vi "AppliedMotionDriveParams.vi"(4 "queue out":refnum<queue>, 6 "user event out":refnum<user-event>, 8 "error in (no error)":errorcluster, 11 "AppliedMotionDrive.lvclass":refnum<class "AppliedMotionDrive.lvclass">) -> (0 "error out":errorcluster, 3 "AppliedMotionDrive.lvclass Out":refnum<class "AppliedMotionDrive.lvclass">)   [LabVIEW 2019, in "AppliedMotionDrive.lvclass"]
doc: "Ce VI est une interface utilisateur qui permet à l'usager d'interagir avec le contrôlleur de moteur ST5-Q"
uses:
  AppliedMotionDrive.lvclass
  C:/Programmes Labview/LabscanV1A/DevicesClass/BaseDevice/BaseDevice.lvclass
  <vilib>/Utility/error.llb/DialogType.ctl
  AppliedMotionDrive.lvclass/AppliedMotionDrive.ctl
panel:
  in  "Update Instr":bool
  in  "Save Act":bool
  in  "LoadAct":bool
  in  "Actuator Settings":u16(ring) items=["Sample Wheel", "Photolum Height", "Filter Wheel"]
  in  "Units":u16(ring) items=["mm", "deg", "pas", "holes"]
  out "Instrument Name":string
  in  "Init":bool
  out "CW Limit":bool
  out "CCW Limit":bool
  out "Alarme":u32
  in  "Update":bool
  in  "Clr Alarm":bool
  out "Status":T1
  in  "Résolution Pas":dbl
  in  "Facteur Dir":bool
  in  "Facteur Pas":dbl=1500.0
  in  "Save":bool
  in  "Accél Max":dbl=0.167 caption="Accélération Max (Tour/s/s)" min=0.167 max=5461.167 step=0.167 format="%#.3g"
  in  "Stop":bool
  in  "Relatif":bool=TRUE caption="Relatif/Absolu\n(Absolu)"
  in  "Origine":bool
  in  "Direction":bool=TRUE
  in  "Déplacement":dbl caption="Position (holes)" min=-2000.0 max=2000.0 step=0.0001 format="%#.3g"
  in  "Décél":dbl=0.167 caption="Décélération \n(Tour/s/s)" min=0.167 max=5461.167 step=0.167 format="%#.3g"
  in  "Accél":dbl=0.167 caption="Accélération \n(Tour/s/s)" min=0.167 max=5461.167 step=0.167 format="%#.3g"
  out "Réponse":string
  in  "Commande":string
  out "Port COM":refnum<visa-resource-name>="COM4"
  in  "Envoyer":bool
  in  "Vitesse":dbl=0.08399999999999999 caption="Vitesse (Tour/s)" min=0.0042 max=133.3333 step=0.0042 format="%#.4g"
  in  "Quitter":bool
  # "Paramètres du moteur"
  # "Contrôle du moteur"
  # "Commande Manuel"
  # "Relatif"
  # "Absolu"
  # "Descendre(H)"
  # "Monter (AH)"
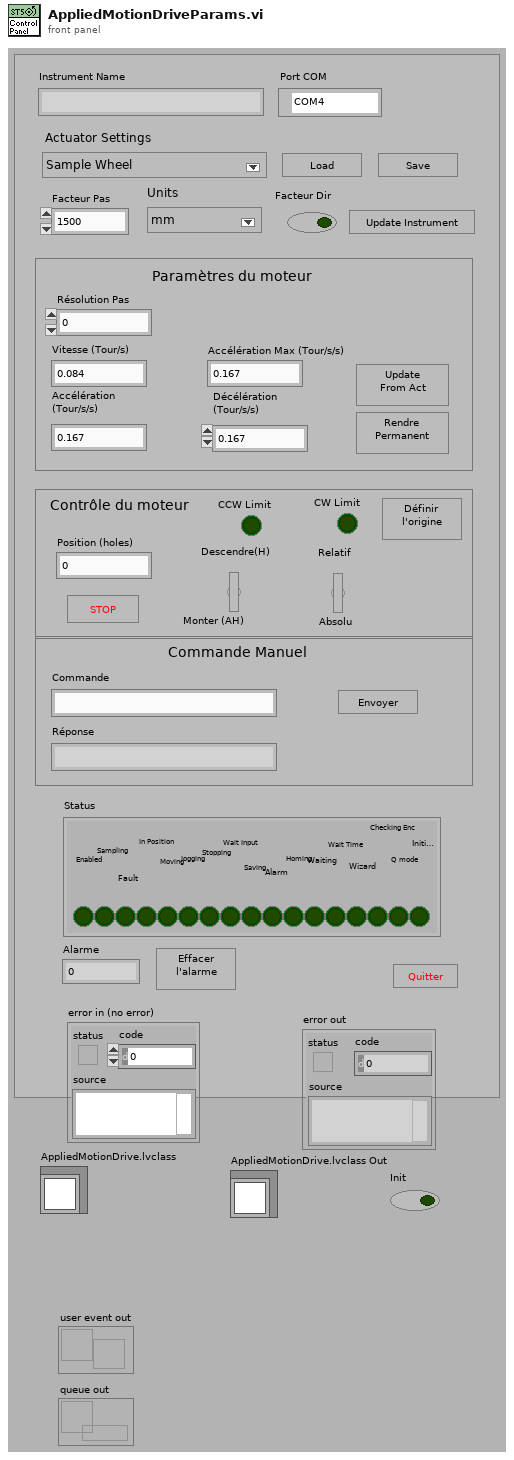
[diagram p1: front panel]
types:
  T1 = cluster{"Enabled":bool, "Sampling":bool, "Fault":bool, "In Position":bool, "Moving":bool, "Jogging":bool, "Stopping":bool, "Wait Input":bool, "Saving":bool, "Alarm":bool, "Homing":bool, "Waiting":bool, "Wait Time":bool, "Wizard":bool, "Checking Enc":bool, "Q mode":bool, "Initializing":bool}
  T2 = enum32{"Invalid", "Standard", "Closed", "Hidden", "Minimized", "Maximized"}
  T3 = typedef "DialogType.ctl" = u16
  T4 = cluster{"Vitesse (Tour/s)":dbl, "Accél":dbl, "Décél":dbl, "Accél Max":dbl, "Idle Current (A) ":dbl}
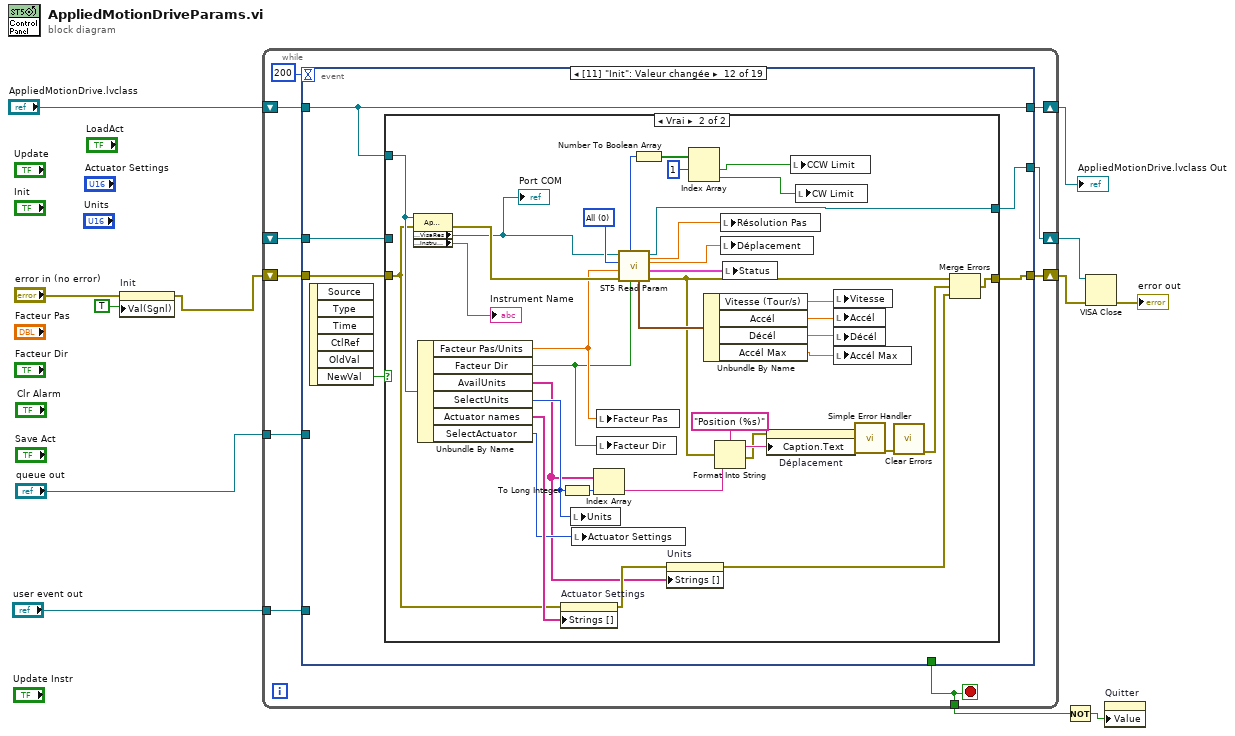
[diagram p0: block diagram]
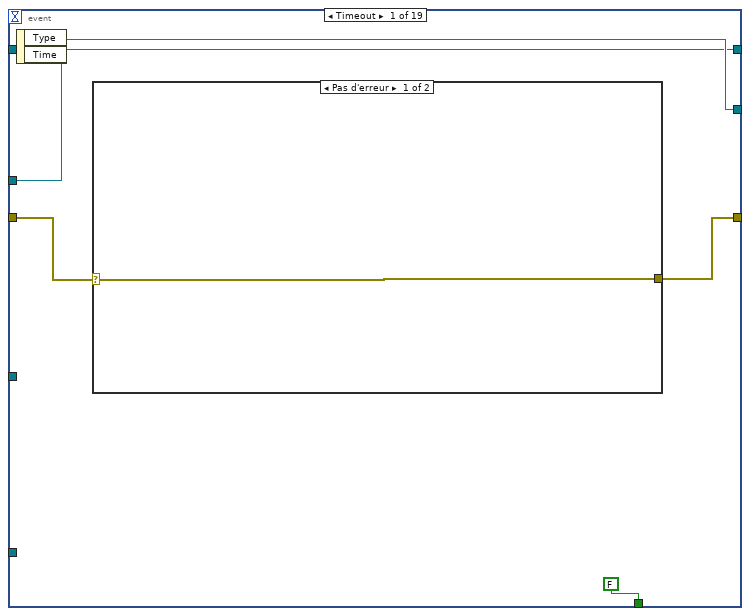
[diagram p2: hidden frame]
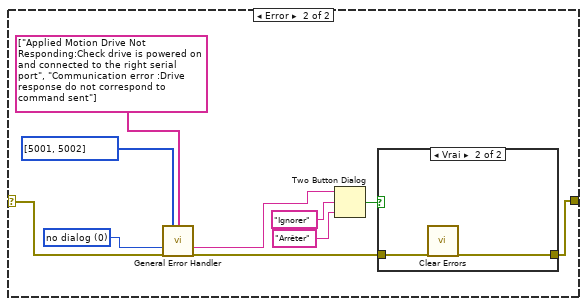
[diagram p3: hidden frame]
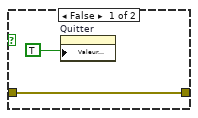
[diagram p4: hidden frame]
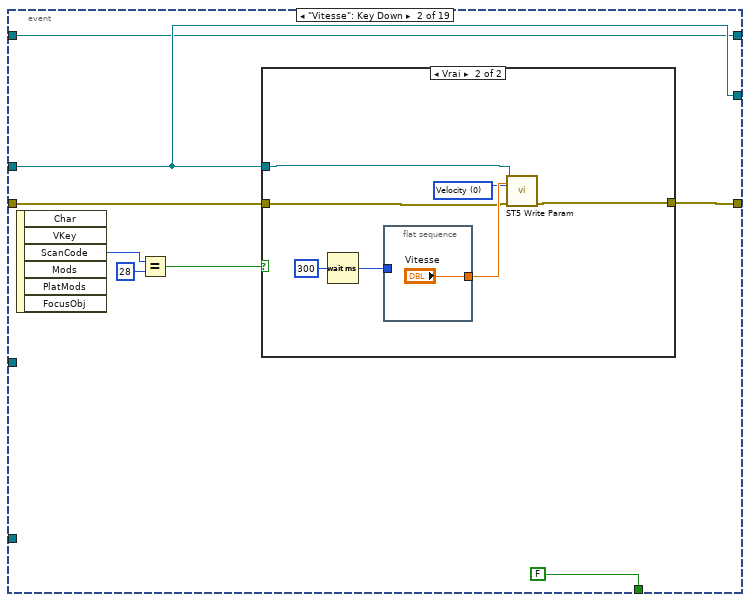
[diagram p5: hidden frame]
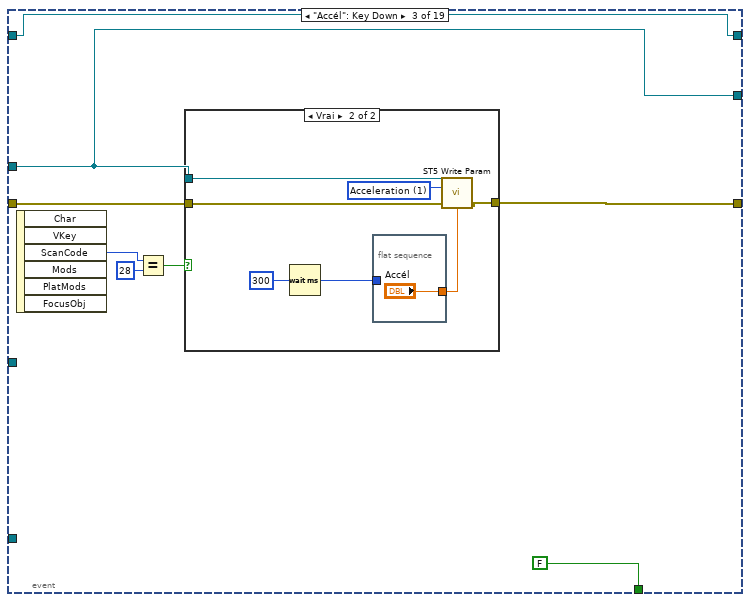
[diagram p7: hidden frame]
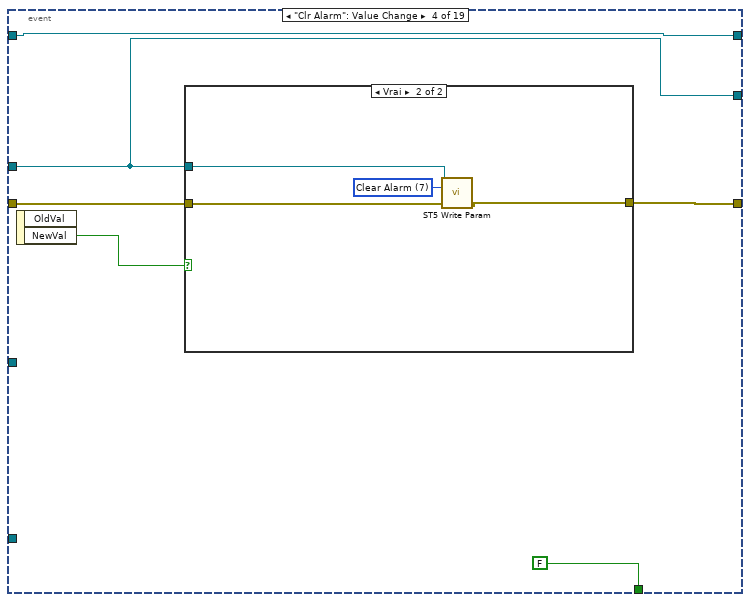
[diagram p9: hidden frame]
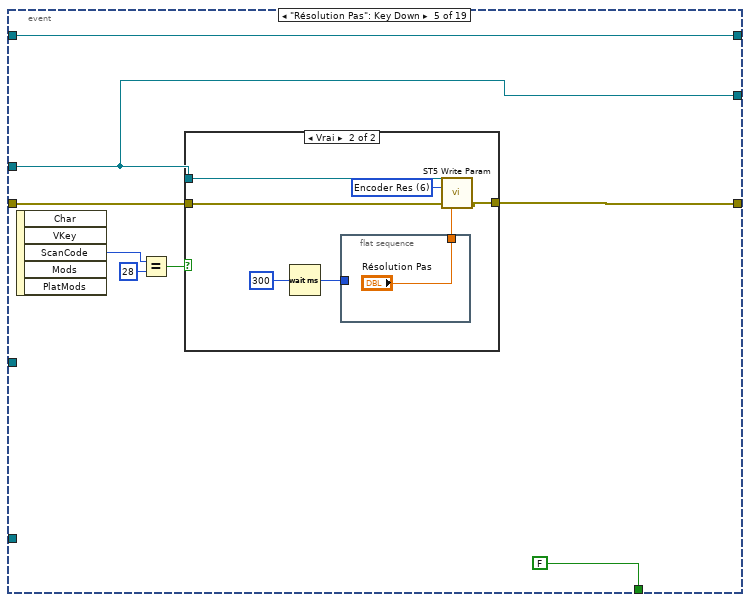
[diagram p11: hidden frame]
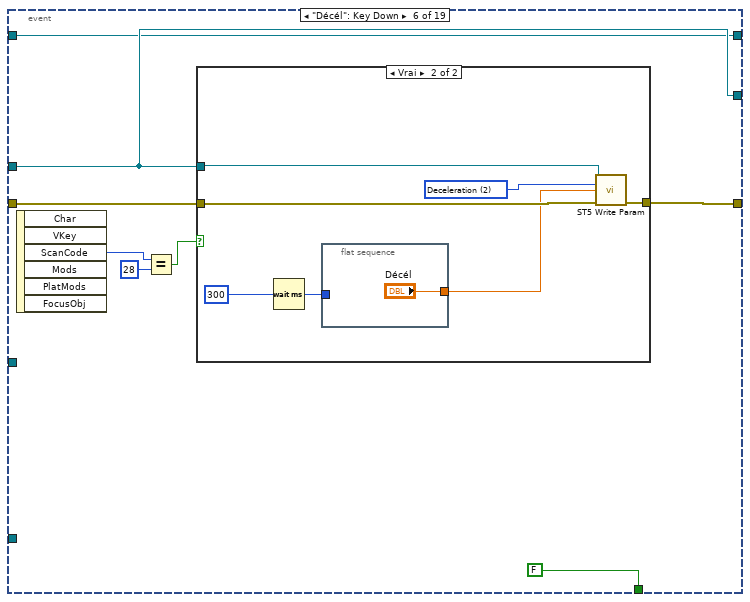
[diagram p13: hidden frame]
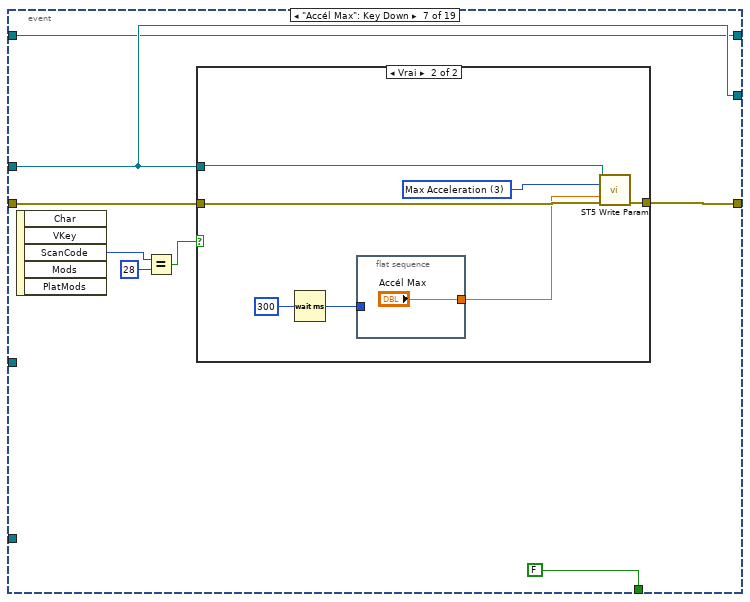
[diagram p15: hidden frame]
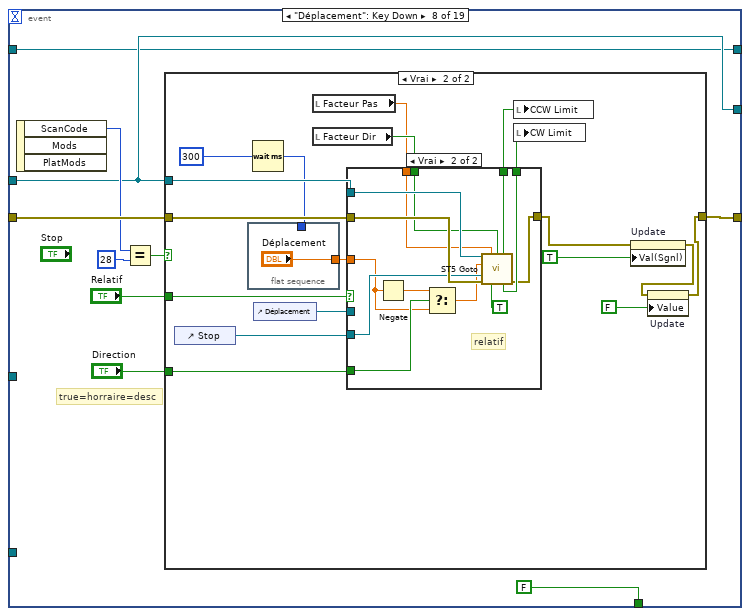
[diagram p17: hidden frame]
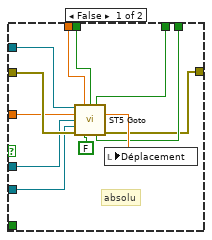
[diagram p19: hidden frame]
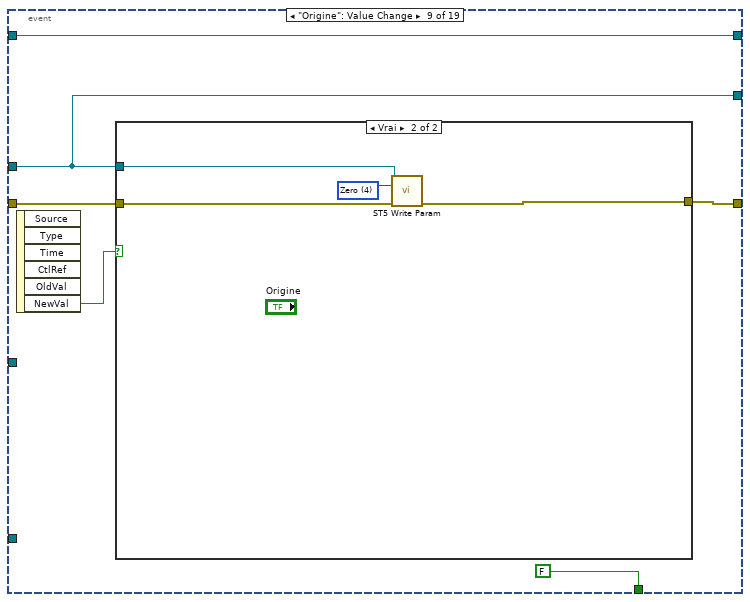
[diagram p20: hidden frame]
diagram:
  n1 = property on="Init" class="Bool (strict)"(error in="error in (no error)", "Val(Sgnl)"=TRUE ("Valeur (Signalisation)")) -> (error out=w5:errorcluster)  [unwired: 1 in, 1 out]
  n2 = while {
    shift-right: [w21] -> w11
    shift-left: w5 -> [w22]
    tunnel: [w18] -> w12
    shift-right: [w17] -> w7
    shift-left: _ -> [w19]
    shift-right: [w15] -> w4
    shift-left: "AppliedMotionDrive.lvclass" -> [w16]
    tunnel: "queue out" -> [w14]
    tunnel: "user event out" -> [w13]
    stop <- w18 stop-if-true
    n3 = event shown="[11] \"Init\": Valeur changée" {
      selector: _ -> [_ _ _ _ _ _ _ _ _ _ _ _ _ _ _ _ _ _ _]
      dyn-events: _ -> [_ _ _ _ _ _ _ _ _ _ _ _ _ _ _ _ _ _ _]
      timeout: 200 -> [_ _ _ _ _ _ _ _ _ _ _ _ _ _ _ _ _ _ _]
      tunnel: w22 -> [w27 w48 w65 w82 w95 w110 w127 w146 w199 w208 w218 w244 w290 w314 w336 w357 _ _ _]
      tunnel: [w26 w47 w64 w81 w94 w109 w126 w145 w198 w207 w217 w243 w289 w313 w335 w356 _ _ _] -> w21
      tunnel: w19 -> [w24 w45 w62 w78 w90 w106 w123 w140 w195 w206 w216 w242 w288 w312 w337 w354 w367 w372 w378]
      tunnel: [FALSE ("Discard?") FALSE ("Discard?") FALSE ("Discard?") FALSE ("Discard?") FALSE ("Discard?") FALSE ("Discard?") FALSE ("Discard?") FALSE ("Discard?") FALSE ("Discard?") _ _ _ _ _ _ FALSE ("Discard?") TRUE ("Discard?") w369 TRUE ("Discard?")] -> w18
      tunnel: [w24 w45 w62 w78 w90 w106 w123 w140 w195 w206 w216 w241 w288 w312 w337 w354 w367 w372 w378] -> w17
      tunnel: w16 -> [w23 w43 w60 w77 w88 w105 w122 w139 w194 w205 w215 w240 w287 w315 w338 w353 w366 w371 w379]
      tunnel: [w23 w43 w60 w77 w88 w105 w122 w139 w194 w205 w215 w240 w286 w315 w338 w353 w366 w371 w379] -> w15
      tunnel: w14 -> [_ _ _ _ _ _ _ _ _ _ _ _ w292 _ _ _ _ _ _]
      tunnel: w13 -> [_ _ _ _ _ _ _ _ _ _ _ _ w291 _ _ _ _ _ _]
      event Timeout {
        n4 = event-data() -> ()  [unwired: 1 in, 2 out]
        n5 = case shown="Pas d'erreur" w27 {
          selector: w27 -> [w28 w32]
          tunnel: [w28 w33] -> w26
          frame No Error {
          }
          frame Error {
            w35 = T3 0 items=["no dialog", "OK message", "continue or stop message", "OK message + warnings", "continue/stop + warnings"] ("type of dialog (OK msg:1)")
            n6 = call <vilib>:"General Error Handler.vi"("[user-defined codes]"=i32[] [5001, 5002], "[user-defined descriptions]"=string[] ["Applied Motion Drive Not Responding:Check drive is powered on and connected to the right serial port", "Communication error :Drive response do not correspond to command sent"], "type of dialog (OK msg:1)"=w35, "error in (no error)"=w32) -> ("message"=w29:string, "error out"=w34:errorcluster)  [unwired: 7 in, 3 out]
            n7 = Two Button Dialog(message=w29, 1:"Arrêter" ("F button name (\"Cancel\")"), 2:"Ignorer" ("T button name (\"OK\")")) -> (T button?=w38:bool)
            n8 = case shown="Vrai" w38 {
              tunnel: w34 -> [w40 w41]
              tunnel: [w40 w42] -> w33
              frame False {
                n9 = property on="Quitter" class="Bool (strict)"("Valeur (Signalisation)"=TRUE ("Value (Signaling)")) -> ()  [unwired: 2 in, 2 out]
              }
              frame True {
                n10 = call <vilib>:"Clear Errors.vi"("error in (no error)"=w41) -> ("error out"=w42:errorcluster)  [unwired: 5 in, 1 out]
              }
            }
          }
        }
      }
      event "Vitesse": Key Down {
        n11 = event-data() -> ("ScanCode"=w44:i16)  [unwired: 1 in, 5 out]
        n12 = Equal?(x=w44, y=i16 28) -> (x = y?=w49:bool)
        n13 = case shown="Vrai" w49 {
          tunnel: w45 -> [_ w53]
          tunnel: w48 -> [w51 w54]
          tunnel: [w51 w58] -> w47
          frame False {
          }
          frame True {
            w56 = u16 0 items=["Velocity", "Acceleration", "Deceleration", "Max Acceleration", "Zero", "Save"] ("Parameters")
            n14 = Wait (ms)(milliseconds to wait=u32 300 ("attente (ms)")) -> (millisecond timer value=w52:u32)
            n15 = flat-sequence {
              tunnel: ["Vitesse"] -> w57
              tunnel: w52 -> [_]
              frame #0 {
              }
            }
            n16 = call <userlib>:"ST5 Write Param.vi"("Port COM"=w53, "Vitesse"=w57, "Parameters"=w56, "error in (no error)"=w54) -> ("error out"=w58:errorcluster)  [unwired: 10 in, 1 out]
          }
        }
      }
      event "Accél": Key Down {
        n17 = event-data() -> ("ScanCode"=w61:i16)  [unwired: 1 in, 5 out]
        n18 = Equal?(x=w61, y=i16 28) -> (x = y?=w66:bool)
        n19 = case shown="Vrai" w66 {
          tunnel: w62 -> [_ w73]
          tunnel: w65 -> [w68 w75]
          tunnel: [w68 w74] -> w64
          frame False {
          }
          frame True {
            w71 = u16 1 items=["Velocity", "Acceleration", "Deceleration", "Max Acceleration", "Zero", "Save"] ("Parameters")
            n20 = Wait (ms)(milliseconds to wait=u32 300 ("attente (ms)")) -> (millisecond timer value=w69:u32)
            n21 = flat-sequence {
              tunnel: ["Accél"] -> w72
              tunnel: w69 -> [_]
              frame #0 {
              }
            }
            n22 = call <userlib>:"ST5 Write Param.vi"("Port COM"=w73, "Accél"=w72, "Parameters"=w71, "error in (no error)"=w75) -> ("error out"=w74:errorcluster)  [unwired: 10 in, 1 out]
          }
        }
      }
      event "Clr Alarm": Value Change {
        n23 = event-data() -> ("NewVal"=w79:bool)  [unwired: 1 in, 1 out]
        n24 = case shown="Vrai" w79 {
          tunnel: w78 -> [_ w85]
          tunnel: w82 -> [w83 w87]
          tunnel: [w83 w86] -> w81
          frame False {
          }
          frame True {
            w84 = u16 7 items=["Velocity", "Acceleration", "Deceleration", "Max Acceleration", "Zero", "Save", "Encoder Res", "Clear Alarm"] ("Parameters")
            n25 = call <userlib>:"ST5 Write Param.vi"("Port COM"=w85, "Parameters"=w84, "error in (no error)"=w87) -> ("error out"=w86:errorcluster)  [unwired: 11 in, 1 out]
          }
        }
      }
      event "Résolution Pas": Key Down {
        n26 = event-data() -> ("ScanCode"=w89:i16)  [unwired: 1 in, 4 out]
        n27 = Equal?(x=w89, y=i16 28) -> (x = y?=w91:bool)
        n28 = case shown="Vrai" w91 {
          tunnel: w90 -> [_ w101]
          tunnel: w95 -> [w96 w103]
          tunnel: [w96 w102] -> w94
          frame False {
          }
          frame True {
            w98 = u16 6 items=["Velocity", "Acceleration", "Deceleration", "Max Acceleration", "Zero", "Save", "Encoder Res", "Clear Alarm"] ("Parameters")
            n29 = Wait (ms)(milliseconds to wait=u32 300 ("attente (ms)")) -> (millisecond timer value=w99:u32)
            n30 = flat-sequence {
              tunnel: w99 -> [_]
              tunnel: ["Résolution Pas"] -> w97
              frame #0 {
              }
            }
            n31 = call <userlib>:"ST5 Write Param.vi"("Port COM"=w101, "Parameters"=w98, "error in (no error)"=w103, "Microstep Res(Pas/Tour)"=w97) -> ("error out"=w102:errorcluster)  [unwired: 10 in, 1 out]
          }
        }
      }
      event "Décél": Key Down {
        n32 = event-data() -> ("ScanCode"=w107:i16)  [unwired: 1 in, 5 out]
        n33 = Equal?(x=w107, y=i16 28) -> (x = y?=w111:bool)
        n34 = case shown="Vrai" w111 {
          tunnel: w106 -> [_ w119]
          tunnel: w110 -> [w113 w120]
          tunnel: [w113 w118] -> w109
          frame False {
          }
          frame True {
            w117 = u16 2 items=["Velocity", "Acceleration", "Deceleration", "Max Acceleration", "Zero", "Save"] ("Parameters")
            n35 = Wait (ms)(milliseconds to wait=u32 300 ("attente (ms)")) -> (millisecond timer value=w115:u32)
            n36 = flat-sequence {
              tunnel: w115 -> [_]
              tunnel: ["Décél"] -> w114
              frame #0 {
              }
            }
            n37 = call <userlib>:"ST5 Write Param.vi"("Port COM"=w119, "Parameters"=w117, "Décél"=w114, "error in (no error)"=w120) -> ("error out"=w118:errorcluster)  [unwired: 10 in, 1 out]
          }
        }
      }
      event "Accél Max": Key Down {
        n38 = event-data() -> ("ScanCode"=w124:i16)  [unwired: 1 in, 4 out]
        n39 = Equal?(x=w124, y=i16 28) -> (x = y?=w128:bool)
        n40 = case shown="Vrai" w128 {
          tunnel: w123 -> [_ w136]
          tunnel: w127 -> [w130 w137]
          tunnel: [w130 w135] -> w126
          frame False {
          }
          frame True {
            w134 = u16 3 items=["Velocity", "Acceleration", "Deceleration", "Max Acceleration", "Zero", "Save"] ("Parameters")
            n41 = Wait (ms)(milliseconds to wait=u32 300 ("attente (ms)")) -> (millisecond timer value=w131:u32)
            n42 = flat-sequence {
              tunnel: ["Accél Max"] -> w133
              tunnel: w131 -> [_]
              frame #0 {
              }
            }
            n43 = call <userlib>:"ST5 Write Param.vi"("Port COM"=w136, "Parameters"=w134, "Accél Max"=w133, "error in (no error)"=w137) -> ("error out"=w135:errorcluster)  [unwired: 10 in, 1 out]
          }
        }
      }
      event "Déplacement": Key Down {
        # "true=horraire=desc"
        n44 = event-data() -> ("ScanCode"=w142:i16)  [unwired: 1 in, 2 out]
        n45 = Equal?(x=w142, y=i16 28) -> (x = y?=w147:bool)
        n46 = case shown="Vrai" w147 {
          tunnel: w140 -> [_ w166]
          tunnel: w146 -> [w149 w167]
          tunnel: [w149 w150] -> w145
          tunnel: "Direction" -> [_ w165]
          tunnel: "Relatif" -> [_ w164]
          frame False {
          }
          frame True {
            n47 = control-ref of="Stop"() -> (w163:refnum<vi>)
            n48 = flat-sequence {
              tunnel: ["Déplacement"] -> w162
              tunnel: w160 -> [_]
              frame #0 {
              }
            }
            n49 = Wait (ms)(milliseconds to wait=u32 300 ("attente (ms)")) -> (millisecond timer value=w160:u32)
            n50 = control-ref of="Déplacement"() -> (w157:refnum<vi>)
            n51 = local read "Facteur Pas"() -> (w158:dbl)
            n52 = local read "Facteur Dir"() -> (w159:bool)
            n53 = case shown="Vrai" w164 {
              tunnel: [w169 w181] -> w153
              tunnel: w167 -> [w179 w192]
              tunnel: w166 -> [w180 w193]
              tunnel: w165 -> [_ w188]
              tunnel: w163 -> [w176 w191]
              tunnel: w162 -> [w175 w186]
              tunnel: w159 -> [w174 w184]
              tunnel: w158 -> [w173 w185]
              tunnel: w157 -> [w172 _]
              tunnel: [w171 w183] -> w156
              tunnel: [w170 w182] -> w155
              frame False {
                # "absolu"
                n54 = call <userlib>:"ST5 Goto.vi"("Port COM"=w180, "Facteur Pas"=w173, "Facteur Dir"=w174, "Position"=w175, "PositionRef"=w172, "Ext Stop Ref"=w176, "error in (no error)"=w179, "Relatif"=FALSE) -> ("CCW Limit"=w171:bool, "Position Out"=w178:dbl, "CW Limit"=w170:bool, "error out"=w169:errorcluster)  [unwired: 1 in, 3 out]
                n55 = local write "Déplacement"(w178) -> ()
              }
              frame True {
                # "relatif"
                n56 = Negate(x=w186) -> (-x=w187:dbl)
                n57 = Select(t=w187, s=w188, f=w186) -> (s? t:f=w190:dbl)
                n58 = call <userlib>:"ST5 Goto.vi"("Port COM"=w193, "Facteur Pas"=w185, "Facteur Dir"=w184, "Position"=w190, "Ext Stop Ref"=w191, "error in (no error)"=w192, "Relatif"=TRUE) -> ("CCW Limit"=w183:bool, "CW Limit"=w182:bool, "error out"=w181:errorcluster)  [unwired: 2 in, 4 out]
              }
            }
            n59 = local write "CCW Limit"(w156) -> ()
            n60 = local write "CW Limit"(w155) -> ()
            n61 = property on="Update" class="Bool (strict)"(error in=w153, "Val(Sgnl)"=TRUE ("Valeur (Signalisation)")) -> (error out=w151:errorcluster)  [unwired: 1 in, 1 out]
            n62 = property on="Update" class="Bool (strict)"(error in=w151, "Value"=FALSE ("Update")) -> (error out=w150:errorcluster)  [unwired: 1 in, 1 out]
          }
        }
      }
      event "Origine": Value Change {
        n63 = event-data() -> ("NewVal"=w196:bool)  [unwired: 1 in, 5 out]
        n64 = case shown="Vrai" w196 {
          tunnel: w199 -> [w200 w203]
          tunnel: w195 -> [_ w201]
          tunnel: [w200 w204] -> w198
          frame False {
          }
          frame True {
            w202 = u16 4 items=["Velocity", "Acceleration", "Deceleration", "Max Acceleration", "Zero", "Save"] ("Parameters")
            n65 = call <userlib>:"ST5 Write Param.vi"("Port COM"=w201, "Parameters"=w202, "error in (no error)"=w203) -> ("error out"=w204:errorcluster)  [unwired: 11 in, 1 out]
          }
        }
      }
      event "Save": Value Change {
        n66 = event-data() -> ("NewVal"=w209:bool)  [unwired: 1 in, 5 out]
        n67 = case shown="Vrai" w209 {
          tunnel: w206 -> [_ w214]
          tunnel: w208 -> [w210 w213]
          tunnel: [w210 w212] -> w207
          frame False {
          }
          frame True {
            w211 = u16 5 items=["Velocity", "Acceleration", "Deceleration", "Max Acceleration", "Zero", "Save"] ("Parameters")
            n68 = call <userlib>:"ST5 Write Param.vi"("Port COM"=w214, "Parameters"=w211, "error in (no error)"=w213) -> ("error out"=w212:errorcluster)  [unwired: 11 in, 1 out]
          }
        }
      }
      event "Update": Value Change {
        n69 = event-data() -> ("NewVal"=w219:bool)  [unwired: 1 in, 5 out]
        n70 = case shown="Vrai" w219 {
          tunnel: w216 -> [_ w228]
          tunnel: w218 -> [w220 w227]
          tunnel: [w220 w229] -> w217
          frame False {
          }
          frame True {
            w237 = u16 0 items=["All", "Velocity", "Acceleration", "Deceleration", "Max Acceleration", "Position"] ("Parameters")
            n71 = local read "Facteur Pas"() -> (w239:dbl)
            n72 = local read "Facteur Dir"() -> (w238:bool)
            n73 = call <userlib>:"ST5 Read Param.vi"("Facteur Dir"=w238, "error in (no error)"=w227, "Facteur Pas"=w239, "Parameters"=w237, "Port COM"=w228) -> ("error out"=w229:errorcluster, "Status"=→"Status":T1, "Position"=w236:dbl, "Speed Par"=w235:T4, "Résolution Pas"=w230:dbl, "Alarme"=w225:u32)  [unwired: 1 out]
            "Alarme" <- w225
            n74 = Number To Boolean Array(number=w225) -> (Boolean array=w224:bool[])
            n75 = Unbundle By Name(w235) -> ("Vitesse (Tour/s)"=w234:dbl, "Accél"=w233:dbl, "Décél"=w232:dbl, "Accél Max"=w231:dbl)
            n76 = Index Array(array=w224, index #1=1 ("indice")) -> (element #1=→"CCW Limit":bool, element #2=→"CW Limit":bool)  [unwired: 1 in]
            n77 = local write "Résolution Pas"(w230) -> ()
            n78 = local write "Déplacement"(w236) -> ()
            n79 = local write "Vitesse"(w234) -> ()
            n80 = local write "Accél"(w233) -> ()
            n81 = local write "Décél"(w232) -> ()
            n82 = local write "Accél Max"(w231) -> ()
          }
        }
      }
      event "Init": Value Change {
        n83 = event-data() -> ("NewVal"=w245:bool)  [unwired: 1 in, 5 out]
        n84 = case shown="Vrai" w245 {
          tunnel: w242 -> [w246 _]
          tunnel: w244 -> [w247 w251]
          tunnel: [w247 w256] -> w243
          tunnel: w240 -> [_ w270]
          tunnel: [w246 w271] -> w241
          frame False {
          }
          frame True {
            w285 = u16 0 items=["All", "Velocity", "Acceleration", "Deceleration", "Max Acceleration", "Position"] ("Parameters")
            n85 = property class="AppliedMotionDrive.lvclass"(reference=w270, error in=w251) -> (error out=w269:errorcluster, "Accessor:VisaRes"=w265:refnum<visa-resource-name>, "Accessor:InstrumentName"=→"Instrument Name":string)  [unwired: 1 out]
            "Port COM" <- w265
            n86 = Unbundle By Name(w270) -> ("Facteur Pas/Units"=w267:dbl, "Facteur Dir"=w266:bool, "AvailUnits"=w248:string[], "SelectUnits"=w254:u8, "Actuator names"=w253:string[], "SelectActuator"=w249:u8)
            n87 = property on="Actuator Settings" class="MDér (strict)"(error in=w251, "Strings []"=w253) -> (error out=w252:errorcluster)  [unwired: 1 in, 1 out]
            n88 = To Long Integer(number=w254) -> (32bit integer=w264:i32)
            n89 = local write "Units"(w254) -> ()
            n90 = local write "Actuator Settings"(w249) -> ()
            n91 = Index Array(array=w248, index=w264) -> (element=w262:string)
            n92 = local write "Facteur Pas"(w267) -> ()
            n93 = local write "Facteur Dir"(w266) -> ()
            n94 = call <userlib>:"ST5 Read Param.vi"("Facteur Dir"=w266, "error in (no error)"=w269, "Facteur Pas"=w267, "Parameters"=w285, "Port COM"=w265) -> ("error out"=w261:errorcluster, "Status"=w272:T1, "Position"=w284:dbl, "Port COM Out"=w271:refnum<visa-resource-name>, "Speed Par"=w283:T4, "Résolution Pas"=w278:dbl, "Alarme"=w277:u32)
            n95 = Number To Boolean Array(number=w277) -> (Boolean array=w276:bool[])
            n96 = property on="Units" class="MDér (strict)"(error in=w252, "Strings []"=w248) -> (error out=w250:errorcluster)  [unwired: 1 in, 1 out]
            n97 = Index Array(array=w276, index #1=1 ("indice")) -> (element #1=w274:bool, element #2=w273:bool)  [unwired: 1 in]
            n98 = Unbundle By Name(w283) -> ("Vitesse (Tour/s)"=w282:dbl, "Accél"=w281:dbl, "Décél"=w280:dbl, "Accél Max"=w279:dbl)
            n99 = Format Into String(format string="Position (%s)", error in=w261, w262) -> (resulting string=w260:string, error out=w259:errorcluster)  [unwired: 1 in]
            n100 = local write "Résolution Pas"(w278) -> ()
            n101 = local write "Déplacement"(w284) -> ()
            n102 = local write "Status"(w272) -> ()
            n103 = property on="Déplacement" class="NumNb (strict)"(error in=w259, "Caption.Text"=w260) -> (error out=w258:errorcluster)  [unwired: 1 in, 1 out]
            n104 = local write "CCW Limit"(w274) -> ()
            n105 = local write "CW Limit"(w273) -> ()
            n106 = local write "Vitesse"(w282) -> ()
            n107 = local write "Accél"(w281) -> ()
            n108 = local write "Décél"(w280) -> ()
            n109 = local write "Accél Max"(w279) -> ()
            n110 = call <vilib>:"Simple Error Handler.vi"("error in (no error)"=w258) -> ("error out"=w257:errorcluster)  [unwired: 4 in, 4 out]
            n111 = call <vilib>:"Clear Errors.vi"("error in (no error)"=w257) -> ("error out"=w255:errorcluster)  [unwired: 5 in, 1 out]
            n112 = Merge Errors(w261, w255, w250) -> (w256:errorcluster)
          }
        }
      }
      event "Update Instr": Value Change {
        n113 = event-data() -> ("NewVal"=w293:bool)  [unwired: 1 in, 5 out]
        n114 = case shown="Vrai" w293 {
          tunnel: w292 -> [_ w310]
          tunnel: w291 -> [_ w309]
          tunnel: w290 -> [w295 w303]
          tunnel: [w295 w307] -> w289
          tunnel: w287 -> [w294 w302]
          tunnel: [w294 w296] -> w286
          frame False {
          }
          frame True {
            n115 = property on="Actuator Settings" class="MDér (strict)"() -> ("Strings []"=w297:string[])  [unwired: 2 in, 2 out]
            n116 = property on="Units" class="MDér (strict)"() -> ("Strings []"=w299:string[])  [unwired: 2 in, 2 out]
            n117 = local read "Facteur Pas"() -> (w298:dbl)
            n118 = local read "Units"() -> (w301:u16)
            n119 = local read "Facteur Dir"() -> (w300:bool)
            n120 = Bundle By Name(cluster=w302, "Facteur Pas/Units"=w298, "Facteur Dir"=w300, "AvailUnits"=w299, "SelectUnits"=w301, "Actuator names"=w297) -> (w296:refnum<class "AppliedMotionDrive.lvclass">)
            n121 = Bundle By Name(cluster=cluster{"Message":string, "Data":variant, i32} {"Message"="Settings", "Data"=variant, 0} ("element"), "Data"=w296) -> (w305:cluster{"Message":string, "Data":variant, i32})
            n122 = Enqueue Element(queue=w310, element=w305, error in (no error)=w303) -> (queue out=w308:refnum<queue>, error out=w304:errorcluster)  [unwired: 1 in, 1 out]
            n123 = Generate User Event(user event=w309, event data cluster=w308, error in=w304) -> (error out=w307:errorcluster)  [unwired: 1 in, 1 out]
          }
        }
      }
      event "Save Act": Value Change {
        n124 = event-data() -> ("NewVal"=w311:bool)  [unwired: 1 in, 5 out]
        n125 = case shown="Vrai" w311 {
          tunnel: w314 -> [w316 w317]
          tunnel: [w316 w324] -> w313
          frame False {
          }
          frame True {
            n126 = property on="Actuator Settings" class="MDér (strict)"(error in=w317) -> (error out=w323:errorcluster, "RingText.Text"=w322:string)  [unwired: 1 in, 1 out]
            n127 = property on="Actuator Settings" class="MDér (strict)"(error in=w317) -> ("Strings []"=w318:string[])  [unwired: 1 in, 2 out]
            n128 = call <userlib>:"ST5 Settings Mess.vi"("error in (no error)"=w323, "Actuator names"=w318, "Name"=w322) -> ("error out"=w321:errorcluster, "Cancel Out"=w320:bool, "Name Out"=w319:string)  [unwired: 6 in]
            n129 = case shown="Faux" w320 {
              tunnel: [w329 w333] -> w324
              tunnel: w321 -> [w327 w333]
              tunnel: w319 -> [w326 _]
              frame False {
                n130 = local read "Facteur Pas"() -> (w331:dbl)
                n131 = local read "Résolution Pas"() -> (w330:dbl)
                n132 = property on="Units" class="MDér (strict)"() -> ("Strings []"=w325:string[])  [unwired: 2 in, 2 out]
                n133 = local read "Facteur Dir"() -> (w328:bool)
                n134 = local read "Units"() -> (w332:u16)
                n135 = call <userlib>:"ST5 Save Act .vi"("Unit Strings"=w325, "Facteur Dir"=w328, "Units"=w332, "error in (no error)"=w327, "Résolution Pas"=w330, "Facteur Pas"=w331, "Actuator Settings"=w326) -> ("error out"=w329:errorcluster)  [unwired: 4 in]
              }
              frame True {
              }
            }
          }
        }
      }
      event "LoadAct": Value Change {
        n136 = event-data() -> ("NewVal"=w334:bool)  [unwired: 1 in, 5 out]
        n137 = case shown="Vrai" w334 {
          tunnel: w336 -> [w339 w350]
          tunnel: [w339 w344] -> w335
          frame False {
          }
          frame True {
            n138 = property on="Actuator Settings" class="MDér (strict)"(error in=w350) -> (error out=w349:errorcluster, "RingText.Text"=w348:string)  [unwired: 1 in, 1 out]
            n139 = call <userlib>:"ST5 Load Act .vi"("error in (no error)"=w349, "Actuator Settings"=w348) -> ("error out"=w341:errorcluster, "Résolution Pas"=w346:dbl, "Facteur Pas"=w347:dbl, "Actuator names"=w343:string[], "Unit Strings"=w342:string[], "Units"=w351:u16, "Facteur Dir"=w352:bool)  [unwired: 2 in, 1 out]
            n140 = property on="Units" class="MDér (strict)"(error in=w341, "Strings []"=w342) -> (error out=w340:errorcluster)  [unwired: 1 in, 1 out]
            n141 = local write "Units"(w351) -> ()
            n142 = local write "Facteur Dir"(w352) -> ()
            n143 = property on="Actuator Settings" class="MDér (strict)"(error in=w340, "Strings []"=w343) -> (error out=w345:errorcluster)  [unwired: 1 in, 1 out]
            n144 = local write "Facteur Pas"(w347) -> ()
            n145 = property on="Résolution Pas" class="NumNb (strict)"(error in=w345, "Val(Sgnl)"=w346) -> (error out=w344:errorcluster)  [unwired: 1 in, 1 out]
          }
        }
      }
      event "Envoyer": Value Change {
        n146 = event-data() -> ("NewVal"=w358:bool)  [unwired: 1 in]
        n147 = case shown="Vrai" w358 {
          tunnel: w357 -> [w359 w363]
          tunnel: [w359 w361] -> w356
          tunnel: w354 -> [_ w364]
          frame False {
          }
          frame True {
            n148 = call <userlib>:"Commande ST5V2.vi"("error in (no error)"=w363, "Commande"="Commande", "Port COM"=w364) -> ("error out"=w361:errorcluster, "Réponse"=→"Réponse":string)  [unwired: 1 in, 2 out]
          }
        }
      }
      event Panel Close? {
        n149 = event-data() -> ()  [unwired: 1 in, 4 out]
        n150 = event-data("Discard?"=FALSE ("Rejeter ?")) -> ()  [unwired: 1 in, 1 out]
      }
      event "Quitter": Value Change {
        n151 = event-data() -> ("NewVal"=w370:bool)  [unwired: 1 in, 5 out]
        n152 = case shown="Vrai" w370 {
          tunnel: [FALSE ("Discard?") TRUE ("Discard?")] -> w369
          frame False {
          }
          frame True {
            n153 = control-ref of="ce VI"() -> (w375:refnum<vi>)
            n154 = property class="VI"(reference=w375, "FP.State"=T2."Closed" ("Fenêtre face-avant : état")) -> ()  [unwired: 1 in, 2 out]
          }
        }
      }
      event Panel Close {
        n155 = event-data() -> ()  [unwired: 1 in, 4 out]
      }
    }
  }
  "AppliedMotionDrive.lvclass Out" <- w4
  n156 = Not(x=w12) -> (.not. x?=w3:bool)
  n157 = VISA Close(VISA resource name=w7, error in (no error)=w11) -> (error out=→"error out":errorcluster)
  n158 = property on="Quitter" class="Bool (strict)"("Value"=w3) -> ()  [unwired: 2 in, 2 out]
